vi "makeplots(SubVI).vi"(0 "Array":u64[](array[numeric]), 1 "Array 5":u64[](array[numeric]), 2 "Array 2":u64[](array[numeric]), 5 "Array 4":u64[](array[numeric]), 7 "Array 9":dbl[](array[numeric]), 9 "Array 6":u64[](array[numeric]), 12 "Array 7":u64[](array[numeric]), 13 "Array 8":u64[](array[numeric]), 14 "Array 3":u64[](array[numeric])) -> (3 "Mixed Signal Graph 1":cluster{"Present (s)":dbl, "number":u64}[](graph), 4 "Mixed Signal Graph 4":T2(graph), 6 "Mixed Signal Graph 3":cluster{"Present (s)":dbl, "number":u64}[](graph), 8 "Mixed Signal Graph 5":T1(graph), 10 "Mixed Signal Graph 2":cluster{"Present (s)":dbl, "number":u64}[](graph))   [LabVIEW 2021]
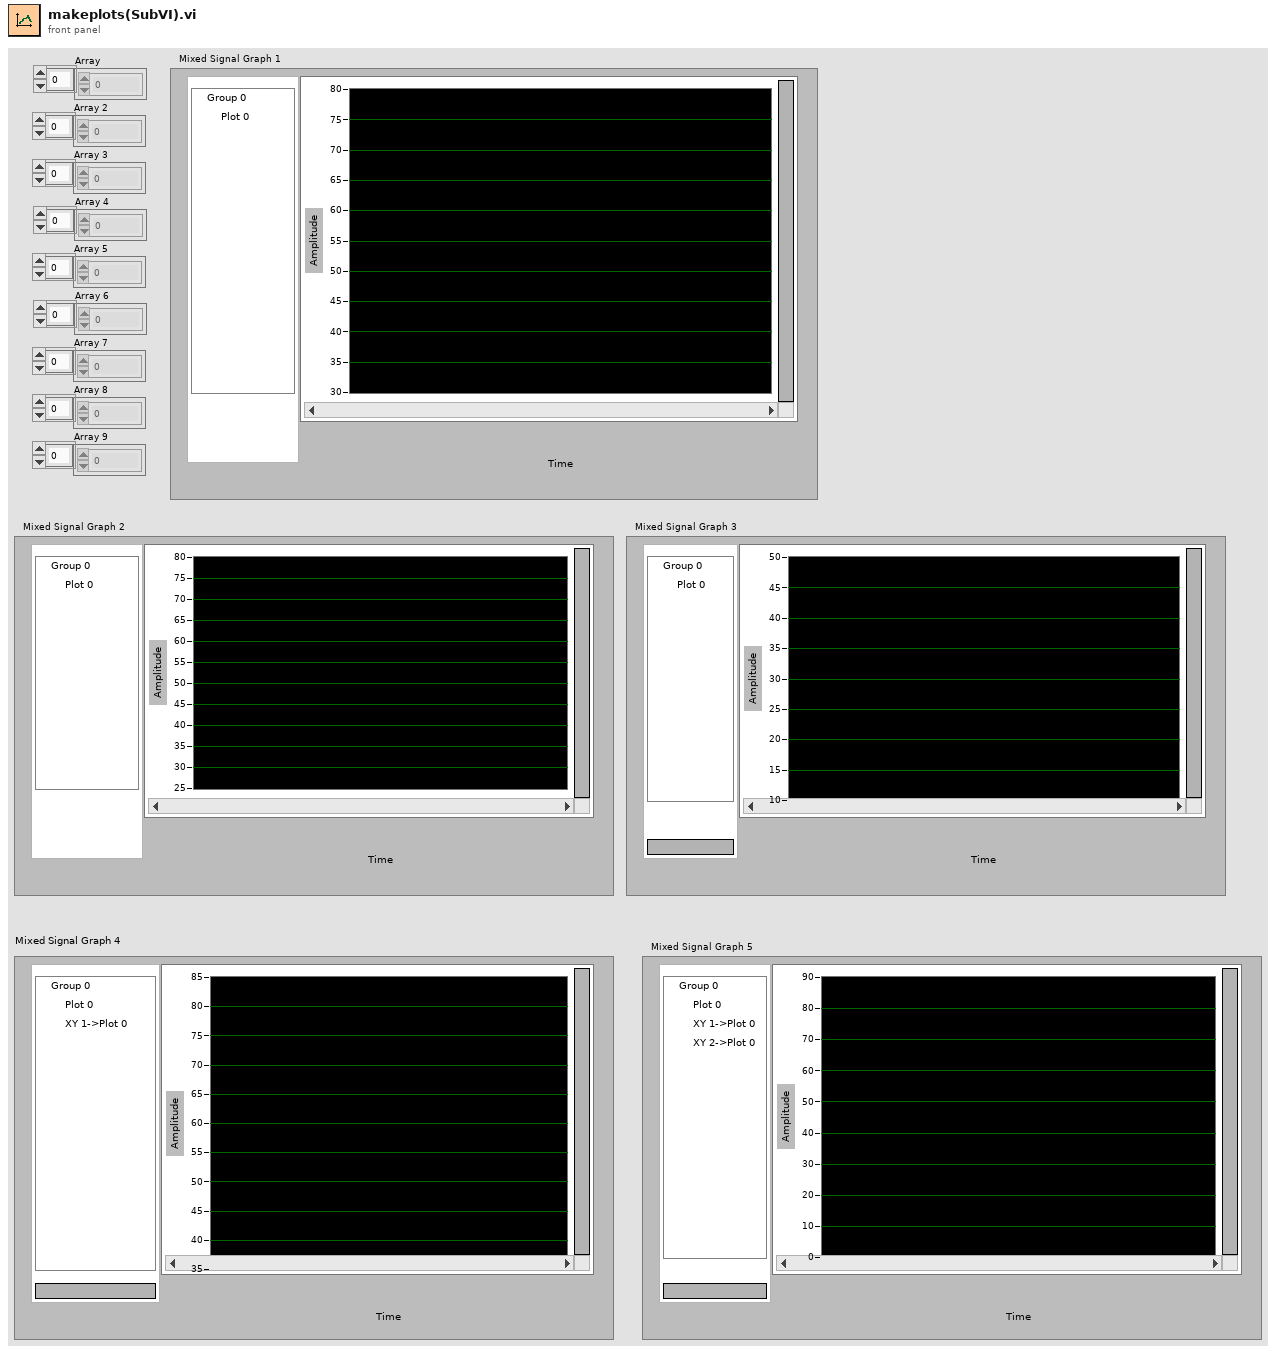
[diagram p1: front panel]
types:
  T1 = cluster{cluster{"Present (s)":dbl, "number":u64}[], cluster{"Present (s)":dbl, "number":u64}[], cluster{"Present (s)":dbl, "number":u64}[]}
  T2 = cluster{cluster{"Present (s)":dbl, "number":u64}[], cluster{"Present (s)":dbl, "number":u64}[]}
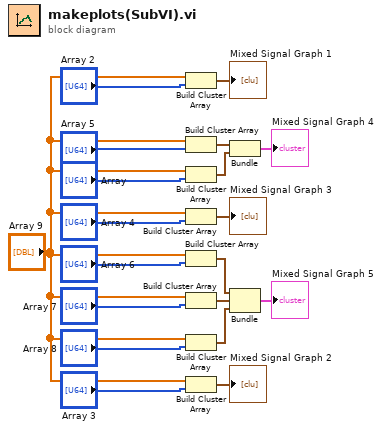
[diagram p0: block diagram]
diagram:
  n1 = Build Cluster Array("Array 9", "Array 2") -> (→"Mixed Signal Graph 1":cluster{"Present (s)":dbl, "number":u64}[])
  n2 = Build Cluster Array("Array 9", "Array 5") -> (w12:cluster{"Present (s)":dbl, "number":u64}[])
  n3 = Build Cluster Array("Array 9", "Array") -> (w17:cluster{"Present (s)":dbl, "number":u64}[])
  n4 = Build Cluster Array("Array 9", "Array 4") -> (→"Mixed Signal Graph 3":cluster{"Present (s)":dbl, "number":u64}[])
  n5 = Build Cluster Array("Array 9", "Array 6") -> (w11:cluster{"Present (s)":dbl, "number":u64}[])
  n6 = Build Cluster Array("Array 9", "Array 7") -> (w16:cluster{"Present (s)":dbl, "number":u64}[])
  n7 = Build Cluster Array("Array 9", "Array 8") -> (w10:cluster{"Present (s)":dbl, "number":u64}[])
  n8 = Build Cluster Array("Array 9", "Array 3") -> (→"Mixed Signal Graph 2":cluster{"Present (s)":dbl, "number":u64}[])
  n9 = Bundle(w12, w17) -> (→"Mixed Signal Graph 4":T2)  [unwired: 1 in]
  n10 = Bundle(w11, w16, w10) -> (→"Mixed Signal Graph 5":T1)  [unwired: 1 in]
